vi "VIGet.vi"(3 "Name":string, 4 "VI Name":string, 5 "Options":i32=16 format="%.0x", 6 "Path":path, 7 "Port":u16=3364, 8 "Address":string="localhost") -> (0 "data string":string, 1 "type string":i16[](array[numeric]), 2 "variant":variant)   [LabVIEW 2014]
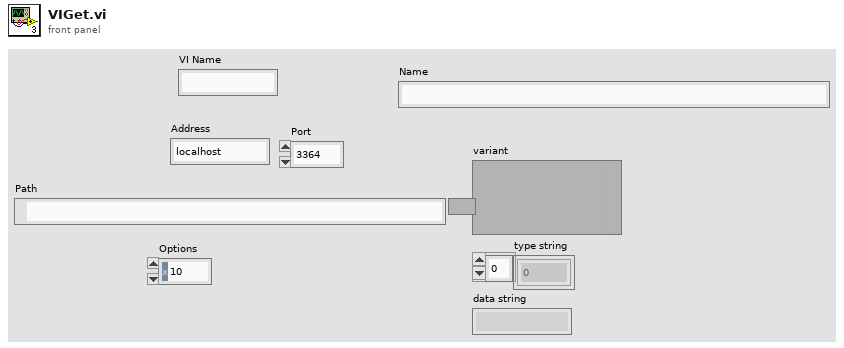
[diagram p1: front panel]
types:
  T1 = cluster{"Name":string, "Reference":refnum<vi>, "Ctrls":cluster{"Name":string, "Ctrl":refnum<vi>}[]}
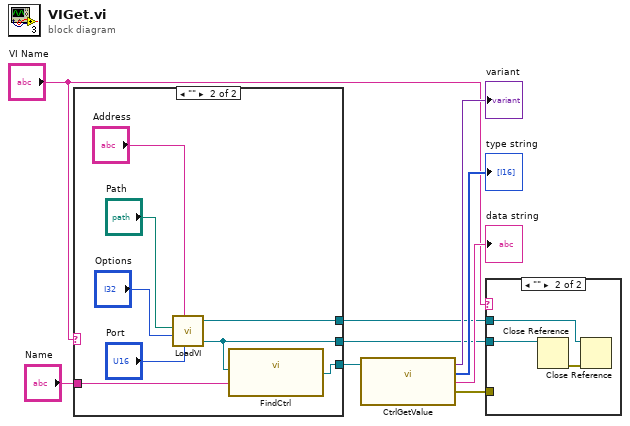
[diagram p0: block diagram]
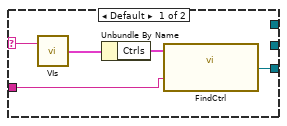
[diagram p3: hidden frame]
diagram:
  n1 = case shown="\"\"" "VI Name" {
    selector: "VI Name" -> [w14 _]
    tunnel: "Name" -> [w11 w21]
    tunnel: [w10 w22] -> w5
    tunnel: [_ w20] -> w3
    tunnel: [_ w17] -> w2
    frame Default {
      n2 = call "VIs.vi"("Name"=w14) -> ("VI Out"=w13:T1)  [unwired: 1 in]
      n3 = Unbundle By Name(w13) -> ("Ctrls"=w12:cluster{"Name":string, "Ctrl":refnum<vi>}[])
      n4 = call "FindCtrl.vi"("Name"=w11, "Ctrls"=w12) -> ("Ctrl"=w10:refnum<vi>)  [unwired: 1 in]
    }
    frame "" {
      n5 = call "LoadVI.vi"("Address"="Address", "Path"="Path", "Options"="Options", "Port"="Port") -> ("LabVIEW Out"=w17:refnum<vi>, "Reference"=w20:refnum<vi>)  [unwired: 3 in]
      n6 = call "FindCtrl.vi"("Name"=w21, "VI"=w20) -> ("Ctrl"=w22:refnum<vi>)  [unwired: 1 in]
    }
  }
  n7 = call "CtrlGetValue.vi"("reference"=w5) -> ("variant"=→"variant":variant, "type string"=→"type string":i16[], "data string"=→"data string":string, "error out"=w1:errorcluster)  [unwired: 1 in]
  n8 = case shown="\"\"" "VI Name" {
    tunnel: w3 -> [_ w25]
    tunnel: w2 -> [_ w23]
    tunnel: w1 -> [_ _]
    frame Default {
    }
    frame "" {
      n9 = Close Reference(reference=w25) -> (error out=w24:errorcluster)  [unwired: 1 in]
      n10 = Close Reference(reference=w23, error in (no error)=w24) -> ()  [unwired: 1 out]
    }
  }
